vi "team_name.vi"(8 "error in (no error)":errorcluster, 11 "PolyVIEW in":refnum<class "PolyVIEW.lvclass">) -> (0 "error out":errorcluster, 2 "teamName":string, 3 "PolyVIEW out":refnum<class "PolyVIEW.lvclass">)   [LabVIEW 2015, in "PolyVIEW.lvclass"]
doc: "Created by Artem Shevelev\nshevelev.pro\nartem@shevelev.pro\nLabVIEW Portal: https://labviewportal.org/memberlist.php?mode=viewprofile&u=2340"
uses:
  PolyVIEW.lvclass
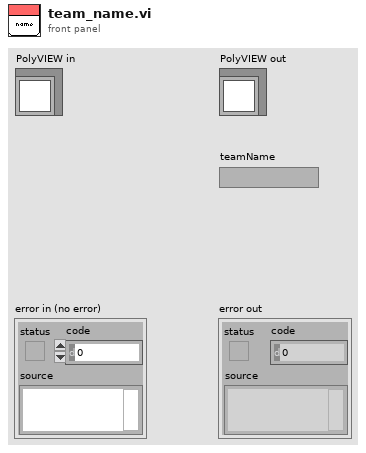
[diagram p1: front panel]
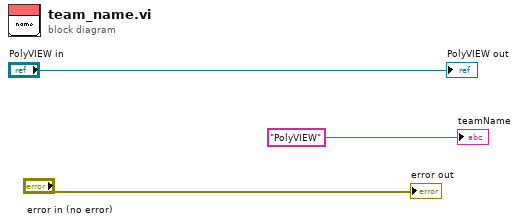
[diagram p0: block diagram]
diagram:
  "error out" <- "error in (no error)"
  "PolyVIEW out" <- "PolyVIEW in"
  "teamName" <- "PolyVIEW" ("teamName")
